vi "Get Parameters.vi"(0 "PF_API in":refnum<class "PF_API.lvclass">, 7 "Parameter Key":string[](array[string]), 9 "Parameter Value":string[](array[string]), 11 "error in (no error)":errorcluster) -> (4 "PF_API out":refnum<class "PF_API.lvclass">, 6 "body":string, 15 "error out":errorcluster)   [LabVIEW 2019, in "PF_API.lvclass"]
uses:
  PF_API.lvclass
  PF_API.lvclass/PF_API.ctl
  <vilib>/httpClient/LabVIEWHTTPClient.lvlib
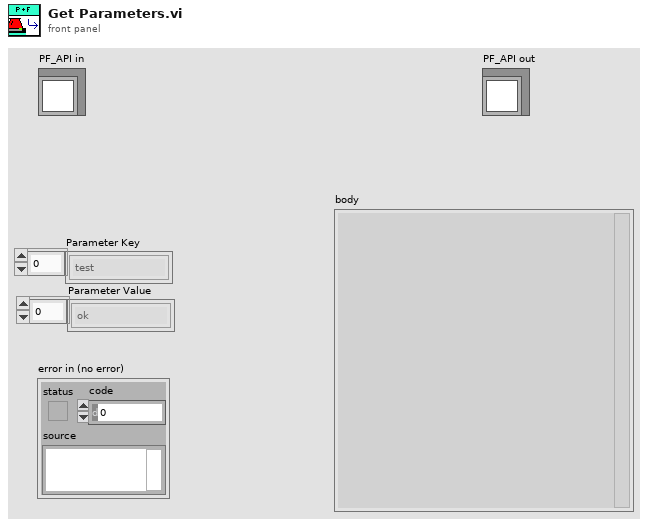
[diagram p1: front panel]
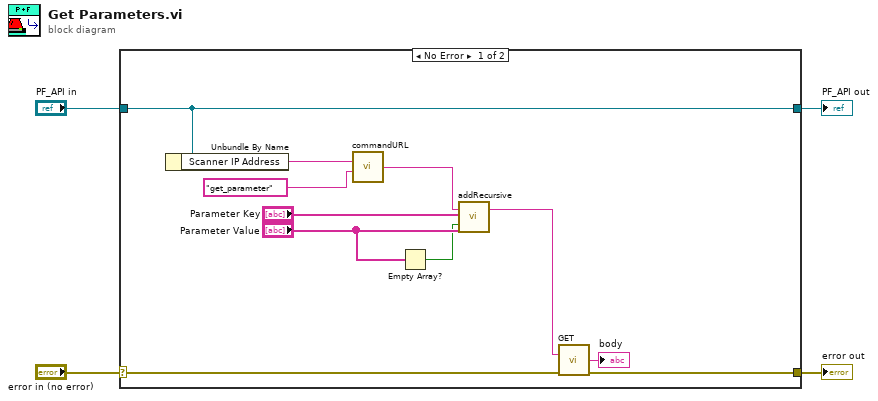
[diagram p0: block diagram]
diagram:
  n1 = case shown="No Error" "error in (no error)" {
    selector: "error in (no error)" -> [w15 w17]
    tunnel: [w11 w17] -> w3
    tunnel: [w14 w16] -> w1
    tunnel: "PF_API in" -> [w14 w16]
    frame No Error {
      n2 = Unbundle By Name(w14) -> ("Scanner IP Address"=w13:string)
      n3 = call "commandURL.vi"("Command String"="get_parameter", "Scanner IP Address"=w13) -> ("Command URL"=w9:string)  [unwired: 4 in]
      n4 = Empty Array?(array="Parameter Value") -> (empty?=w5:bool)
      n5 = call "addRecursive.vi"("Command URL in"=w9, "Parameter Key"="Parameter Key", "Parameter Value"="Parameter Value", "Finish? in"=w5) -> ("Command URL out"=w8:string)  [unwired: 12 in, 3 out]
      n6 = call <vilib>:"GET.vi"("url"=w8, "error in (no error)"=w15) -> ("body"=→"body":string, "error out"=w11:errorcluster)  [unwired: 10 in, 2 out]
    }
    frame Error {
    }
  }
  "error out" <- w3
  "PF_API out" <- w1
